vi "coordinates.vi"(0 "read buffer":string="X0,Y0,Z0\r\n") -> (1 "Current coordinates":T1, 2 "Current coordinates":cluster{"X":dbl, "Y":dbl, "Z":dbl})   [LabVIEW 2018]
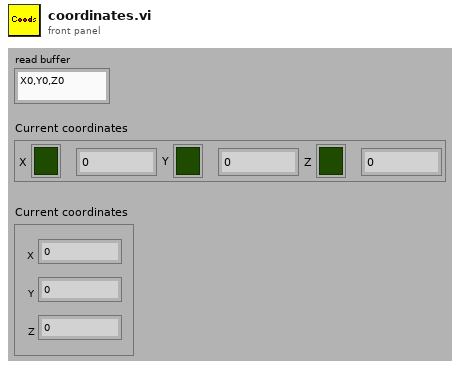
[diagram p1: front panel]
types:
  T1 = cluster{"Steps":dbl, "X":bool, "Steps 2":dbl, "Y":bool, "Steps 3":dbl, "Z":bool}
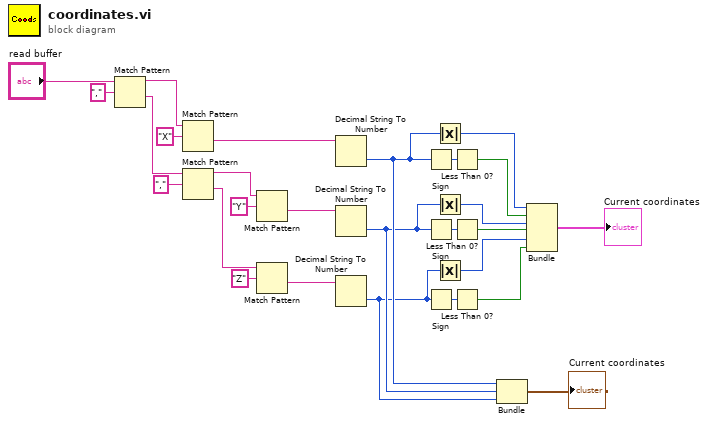
[diagram p0: block diagram]
diagram:
  n1 = Match Pattern(string="read buffer", regular expression=",") -> (before substring=w24:string, after substring=w20:string)  [unwired: 1 in, 2 out]
  n2 = Match Pattern(string=w24, regular expression="X") -> (after substring=w17:string)  [unwired: 1 in, 3 out]
  n3 = Match Pattern(string=w20, regular expression=",") -> (before substring=w21:string, after substring=w18:string)  [unwired: 1 in, 2 out]
  n4 = Match Pattern(string=w21, regular expression="Y") -> (after substring=w16:string)  [unwired: 1 in, 3 out]
  n5 = Match Pattern(string=w18, regular expression="Z") -> (after substring=w15:string)  [unwired: 1 in, 3 out]
  n6 = Decimal String To Number(string=w17) -> (number=w4:i32)  [unwired: 2 in, 1 out]
  n7 = Decimal String To Number(string=w16) -> (number=w3:i32)  [unwired: 2 in, 1 out]
  n8 = Decimal String To Number(string=w15) -> (number=w2:i32)  [unwired: 2 in, 1 out]
  n9 = Sign(1:w4) -> (0:w14:i32)
  n10 = Sign(1:w3) -> (0:w13:i32)
  n11 = Sign(1:w2) -> (0:w12:i32)
  n12 = Absolute Value(x=w4) -> (abs(x)=w7:i32)
  n13 = Absolute Value(x=w3) -> (abs(x)=w6:i32)
  n14 = Absolute Value(x=w2) -> (abs(x)=w5:i32)
  n15 = Less Than 0?(x=w14) -> (x < 0?=w11:bool)
  n16 = Less Than 0?(x=w13) -> (x < 0?=w10:bool)
  n17 = Less Than 0?(x=w12) -> (x < 0?=w9:bool)
  n18 = Bundle(w4, w3, w2) -> (→"Current coordinates":cluster{i32, i32, i32})  [unwired: 1 in]
  n19 = Bundle(w7, w11, w6, w10, w5, w9) -> (→"Current coordinates":cluster{i32, bool, i32, bool, i32, bool})  [unwired: 1 in]
